vi "Evaporation Rate.vi"(11 "array":dbl[](array[numeric])) -> (3 "Evaporation Rate":dbl)   [LabVIEW 2020]
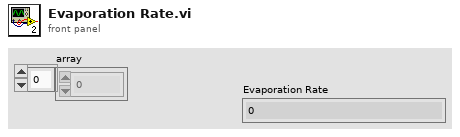
[diagram p1: front panel]
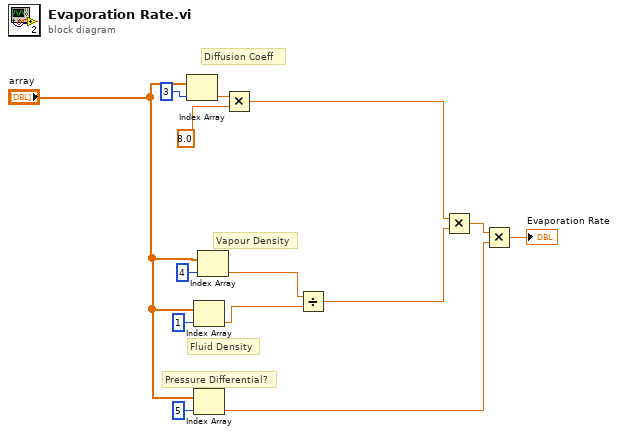
[diagram p0: block diagram]
diagram:
  # "Pressure Differential?"
  # "Diffusion Coeff"
  # "Fluid Density"
  # "Vapour Density"
  n1 = Index Array(array="array", index=3) -> (element=w14:dbl)
  n2 = Index Array(array="array", index=1) -> (element=w9:dbl)
  n3 = Index Array(array="array", index=5) -> (element=w4:dbl)
  n4 = Index Array(array="array", index=4) -> (element=w10:dbl)
  n5 = Multiply(x=w14, y=8.0) -> (x*y=w8:dbl)
  n6 = Divide(x=w10, y=w9) -> (x/y=w7:dbl)
  n7 = Multiply(x=w8, y=w7) -> (x*y=w6:dbl)
  n8 = Multiply(x=w6, y=w4) -> (x*y=→"Evaporation Rate":dbl)
